vi "ff_read_loop_test.vi"() -> ()   [LabVIEW 2016]
uses:
  FF/FF_Read(polymorphic).llb/FF_Read(float).vi
panel:
  out "Array":sgl[](array[numeric])
  in  "stop":bool
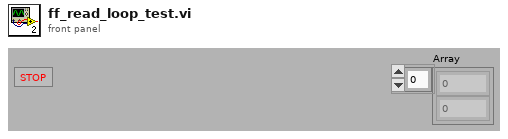
[diagram p1: front panel]
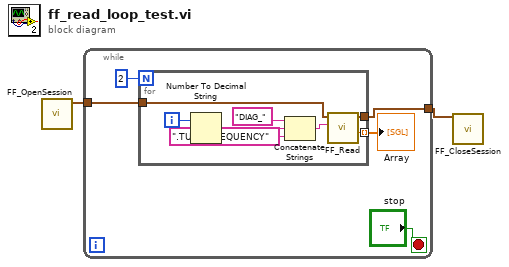
[diagram p0: block diagram]
diagram:
  n1 = call "FF_OpenSession.vi"() -> ("refnum out"=w2:cluster{"Handle1":u32, "Handle2":u32})  [unwired: 10 in, 1 out]
  n2 = while {
    tunnel: w2 -> [w6]
    tunnel: [w3] -> w1
    stop <- "stop" stop-if-true
    n3 = for {
      N: 2 -> [_]
      tunnel: w6 -> [w15]
      tunnel: [w9] -> w4 mode=indexing
      tunnel: [w8] -> w3
      i -> [w12]
      n4 = Number To Decimal String(number=w12) -> (decimal integer string=w11:string)  [unwired: 1 in]
      n5 = Concatenate Strings("DIAG_" ("tag"), w11, ".TUBE_FREQUENCY" ("string")) -> (w13:string)
      n6 = call-poly "FF_Read.vi"("tag"=w13, "refnum in"=w15) -> ("value"=w9:sgl, "refnum out"=w8:cluster{"Handle1":u32, "Handle2":u32})  [unwired: 7 in, 1 out]
    }
    "Array" <- w4
  }
  n7 = call "FF_CloseSession.vi"("refnum in"=w1) -> ()  [unwired: 10 in, 1 out]
